vi "SetIntakeSpeed.vi"(8 "error in":errorcluster, 11 "Speed":dbl) -> (0 "error out":errorcluster)   [LabVIEW 2016]
doc: "Sets intake speed global variable"
uses:
  Robot Global Data.vi
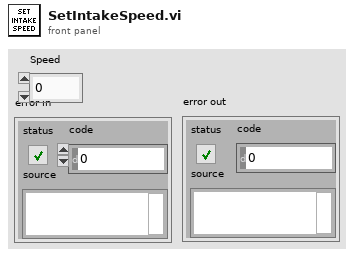
[diagram p1: front panel]
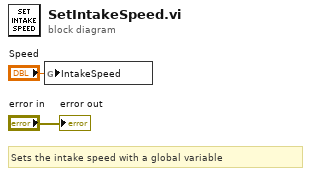
[diagram p0: block diagram]
diagram:
  # "Sets the intake speed with a global variable"
  n1 = global write "Robot Global Data.vi" "IntakeSpeed"("Speed") -> ()
  "error out" <- "error in"
